vi "LoadImageFile.vi"(8 "error in (no error)":errorcluster, 9 "mode":i32(ring) items=["Rgb", "Greyscale"], 10 "FilePath":path, 11 "FaceRecognition in":refnum<class "FaceRecognition.lvclass">) -> (0 "error out":errorcluster, 2 "LoadImageFile":refnum<k24>, 3 "FaceRecognition out":refnum<class "FaceRecognition.lvclass">)   [LabVIEW 2020, in "FaceRecognitionDotNet.lvlib" / "FaceRecognition.lvclass"]
uses:
  FaceRecognition.lvclass
  dll/FaceRecognitionDotNet.dll
  FaceRecognition.lvclass/FaceRecognition.ctl
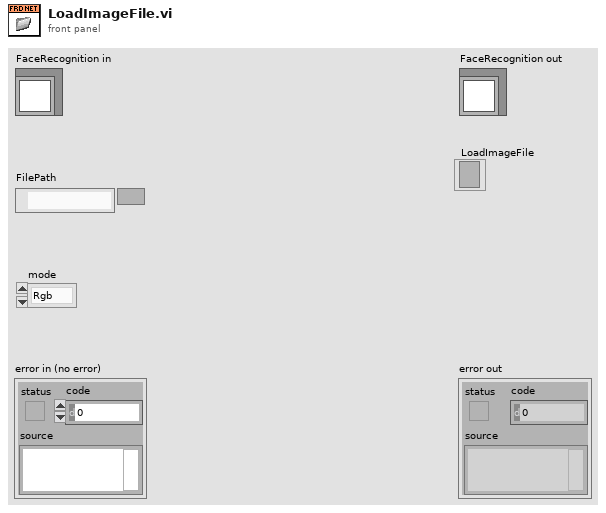
[diagram p1: front panel]
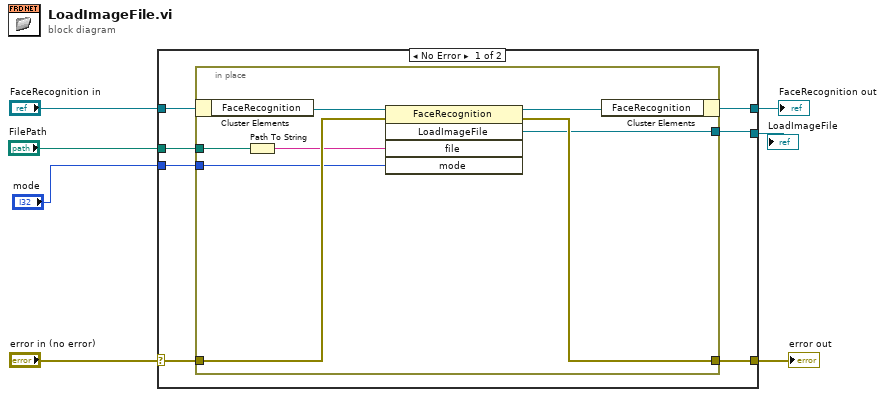
[diagram p0: block diagram]
diagram:
  n1 = case shown="No Error" "error in (no error)" {
    selector: "error in (no error)" -> [w12 w24]
    tunnel: [w11 w24] -> w6
    tunnel: [w13 w23] -> w4
    tunnel: "FaceRecognition in" -> [w14 w23]
    tunnel: [w10 _] -> w3
    tunnel: "FilePath" -> [w9 _]
    tunnel: "mode" -> [w8 _]
    frame No Error {
      n2 = in-place {
        in-place-border: w12 -> [w20]
        in-place-border: [w19] -> w11
        in-place-border: [w18] -> w10
        in-place-border: w9 -> [w16]
        in-place-border: w8 -> [w15]
        n3 = in-place-cluster #1(w14) -> ("FaceRecognition"=w22:refnum<k24>)
        n4 = Path To String(path=w16) -> (string=w17:string)
        n5 = invoke class="FaceRecognition" method="LoadImageFile"(reference=w22, error in=w20, "file"=w17, "mode"=w15) -> (reference out=w21:refnum<k24>, error out=w19:errorcluster, "LoadImageFile"=w18:refnum<k24>)  [unwired: 1 in, 2 out]
        n6 = in-place-cluster #1("FaceRecognition"=w21) -> (w13:refnum<class "FaceRecognition.lvclass">)
      }
    }
    frame Error {
    }
  }
  "error out" <- w6
  "FaceRecognition out" <- w4
  "LoadImageFile" <- w3
